vi "OAT Frequency Shift (Mixer).vi"(6 "initial phase":dbl format="%.2f", 10 "fc":dbl format="%.2f", 11 "X":dbl[](array[numeric]) format="%.2f") -> (2 "imaginary":dbl[](array[numeric]) format="%.2f", 3 "real":dbl[](array[numeric]) format="%.2f", 4 "final phase":dbl format="%.2f")   [LabVIEW 2017, in "SoundVib_Resampling.lvlib"]
uses:
  <vilib>/addons/Sound and Vibration/Order Analysis/Resample Order Tracking/SoundVib_Resampling.lvlib
  <resource>/sndvib.dll
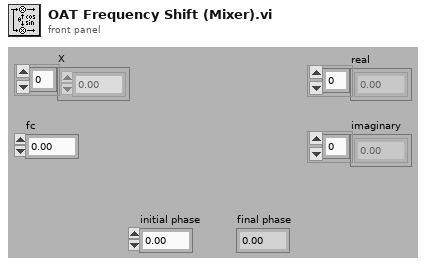
[diagram p1: front panel]
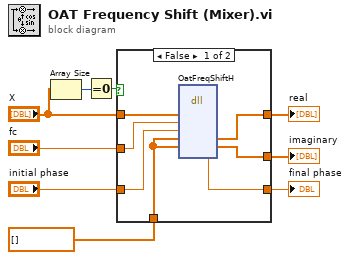
[diagram p0: block diagram]
diagram:
  n1 = Array Size(array="X") -> (size(s)=w2:i32)
  n2 = Equal To 0?(x=w2) -> (x = 0?=w1:bool)
  n3 = case shown="False" w1 {
    tunnel: "initial phase" -> [w16 w17]
    tunnel: "fc" -> [w15 _]
    tunnel: [w14 w18] -> w7
    tunnel: [w13 w18] -> w6
    tunnel: [w12 w17] -> w5
    tunnel: dbl[] [] ("realOutput") -> [w11 _]
    tunnel: "X" -> [w10 w18]
    frame False {
      n4 = dll-call lib="C:/Program Files (x86)/National Instruments/LabVIEW 2017/resource/sndvib.*" fn="OatFreqShiftH"("xH"=w10, "fc"=w15, "initPhase"=w16, "realOutput"=w11, "imagOutput"=w11) -> ("realOutput"=w14:dbl[], "imagOutput"=w13:dbl[], "finalPhase"=w12:dbl)  [unwired: 8 in, 2 out]
    }
    frame True {
    }
  }
  "imaginary" <- w6
  "real" <- w7
  "final phase" <- w5
